vi "FineCalibration.vi"(0 "Connection Cluster in":T1, 2 "Fine Callibration Velocity 2":dbl, 3 "Start Position":dbl, 4 "Fine range":dbl, 5 "Iterations":u32=10) -> (14 "Connection Cluster out":T1, 16 "Peak (right)":dbl, 17 "Peak (left)":dbl)   [LabVIEW 2013]
uses:
  Global.vi
panel:
  out "XY Graph 2":cluster{"Array":dbl[], "Array":dbl[]}(graph)
  out "XY Graph":cluster{"Array":dbl[], "Array":dbl[]}(graph)
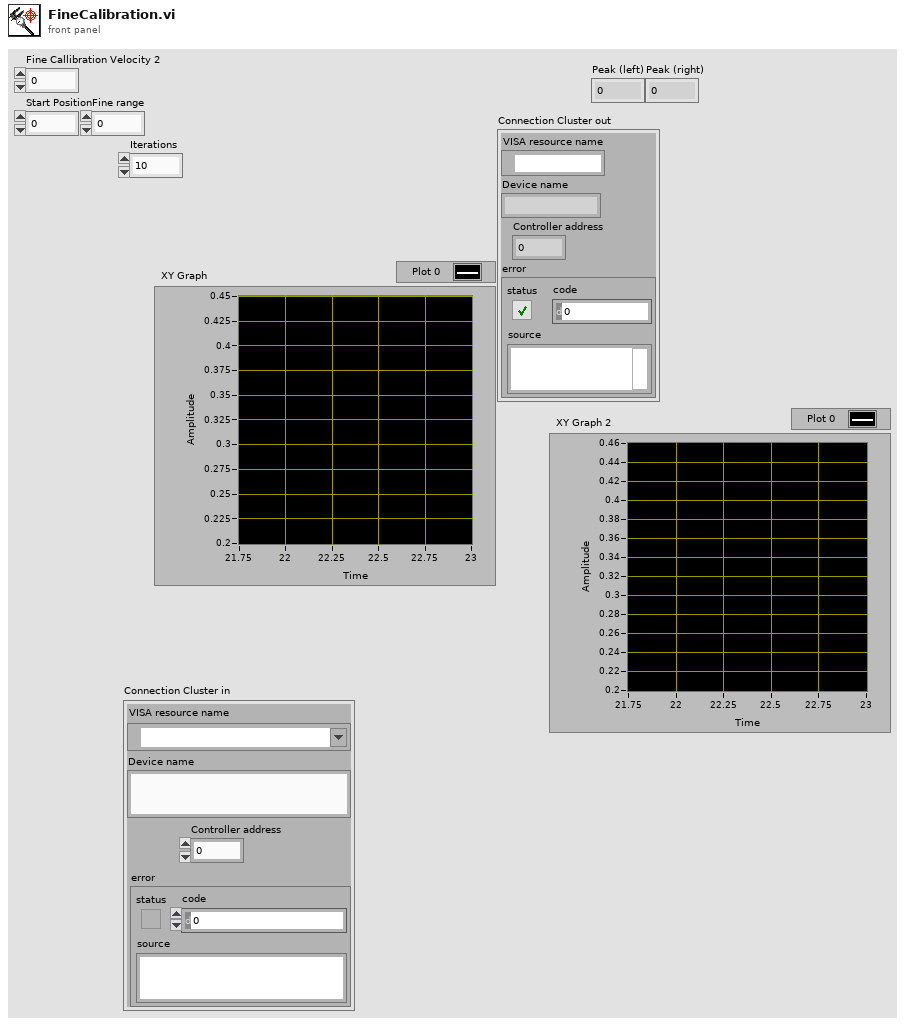
[diagram p1: front panel]
types:
  T1 = cluster{"VISA resource name":refnum<visa-resource-name>, "Device name":string, "Controller address":i32, "error":errorcluster}
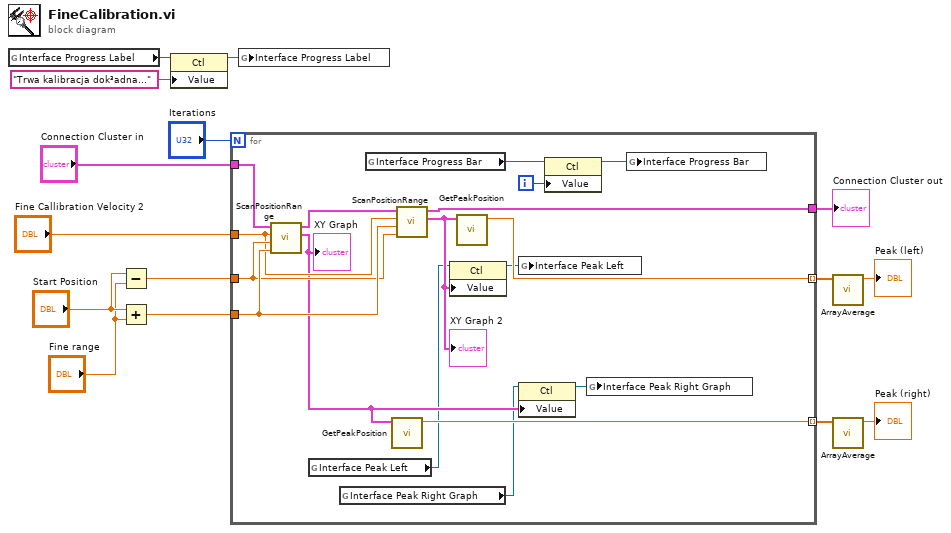
[diagram p0: block diagram]
diagram:
  n1 = global read "Global.vi" "Interface Progress Label"() -> (w2:refnum<vi>)
  n2 = Subtract(x="Start Position", y="Fine range") -> (x-y=w14:dbl)
  n3 = Add(x="Start Position", y="Fine range") -> (x+y=w13:dbl)
  n4 = property class="Ctl"(reference=w2, "Value"="Trwa kalibracja dok³adna...") -> (reference out=w1:refnum<vi>)  [unwired: 1 in, 1 out]
  n5 = for {
    N: "Iterations" -> [_]
    tunnel: "Fine Callibration Velocity 2" -> [w28]
    tunnel: "Connection Cluster in" -> [w31]
    tunnel: w14 -> [w29]
    tunnel: w13 -> [w30]
    tunnel: [w27] -> w10 mode=indexing
    tunnel: [w26] -> w11 mode=indexing
    tunnel: [w25] -> w12
    i -> [w24]
    n6 = call "ScanPositionRange.vi"("Target position"=w30, "Start position"=w29, "Velocity"=w28, "Connection Cluster in"=w31) -> ("output cluster"=w22:cluster{dbl[], dbl[]}, "Connection Cluster out"=w32:T1)  [unwired: 6 in]
    "XY Graph" <- w22
    n7 = global read "Global.vi" "Interface Peak Left"() -> (w21:refnum<vi>)
    n8 = global read "Global.vi" "Interface Peak Right Graph"() -> (w19:refnum<vi>)
    n9 = global read "Global.vi" "Interface Progress Bar"() -> (w17:refnum<vi>)
    n10 = call "GetPeakPosition.vi"("Input cluster"=w22) -> ("Peak position [mm]"=w27:dbl)  [unwired: 10 in]
    n11 = call "ScanPositionRange.vi"("Target position"=w29, "Start position"=w30, "Velocity"=w28, "Connection Cluster in"=w32) -> ("output cluster"=w23:cluster{dbl[], dbl[]}, "Connection Cluster out"=w25:T1)  [unwired: 6 in]
    "XY Graph 2" <- w23
    n12 = property class="Ctl"(reference=w21, "Value"=w23) -> (reference out=w20:refnum<vi>)  [unwired: 1 in, 1 out]
    n13 = call "GetPeakPosition.vi"("Input cluster"=w23) -> ("Peak position [mm]"=w26:dbl)  [unwired: 10 in]
    n14 = global write "Global.vi" "Interface Peak Left"(w20) -> ()
    n15 = property class="Ctl"(reference=w19, "Value"=w22) -> (reference out=w18:refnum<vi>)  [unwired: 1 in, 1 out]
    n16 = property class="Ctl"(reference=w17, "Value"=w24) -> (reference out=w16:refnum<vi>)  [unwired: 1 in, 1 out]
    n17 = global write "Global.vi" "Interface Peak Right Graph"(w18) -> ()
    n18 = global write "Global.vi" "Interface Progress Bar"(w16) -> ()
  }
  "Connection Cluster out" <- w12
  n19 = global write "Global.vi" "Interface Progress Label"(w1) -> ()
  n20 = call "ArrayAverage.vi"("array"=w11) -> ("Average"=→"Peak (left)":dbl)  [unwired: 10 in]
  n21 = call "ArrayAverage.vi"("array"=w10) -> ("Average"=→"Peak (right)":dbl)  [unwired: 10 in]
